vi "demo - cluster intro.vi"() -> ()   [LabVIEW 2023]
panel:
  out "scope output":T1
  in  "scope settings":T1
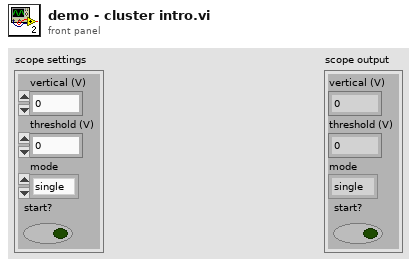
[diagram p1: front panel]
types:
  T1 = cluster{"vertical (V)":dbl, "threshold (V)":dbl, "mode":enum16{"single", "continuous"}, "start?":bool}
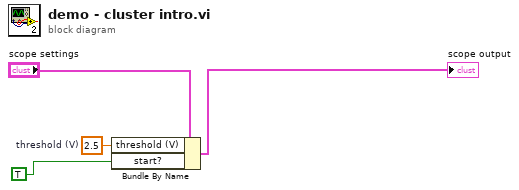
[diagram p0: block diagram]
diagram:
  w3 = 2.5  # threshold (V)
  n1 = Bundle By Name(cluster="scope settings", "threshold (V)"=w3, "start?"=TRUE) -> (→"scope output":T1)
